vi "Define Default Prefix.vi"(8 "error in":errorcluster, 11 "DI channel in":refnum<class "DI Channel.lvclass">) -> (0 "error out":errorcluster, 3 "DI channel out":refnum<class "DI Channel.lvclass">)   [LabVIEW 2020, in "Scan Engine Scripting.lvlib" / "DI Channel.lvclass"]
uses:
  DI Channel.lvclass
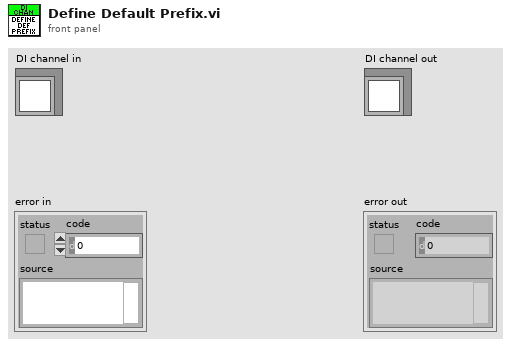
[diagram p1: front panel]
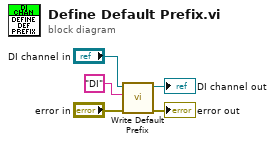
[diagram p0: block diagram]
diagram:
  n1 = call-dynamic "Write Default Prefix.vi"("error in"="error in", "default prefix"="DI", "channel in"="DI channel in") -> ("error out"=→"error out":errorcluster, "channel out"=→"DI channel out":refnum<class "DI Channel.lvclass">)  [unwired: 7 in]
